vi "Make.vi"(8 "error in (no error)":errorcluster, 9 "Item Refnum":refnum<vi>, 10 "Target":refnum<vi>, 11 "Coupled Message Scripter":refnum<class "Coupled Message Scripter.lvclass">) -> (0 "error out":errorcluster, 3 "Coupled Message Scripter out":refnum<class "Coupled Message Scripter.lvclass">)   [LabVIEW 2020, in "Message Maker.lvlib" / "Coupled Message Scripter.lvclass"]
uses:
  Coupled Message Scripter.lvclass
  Coupled Message Scripter.lvclass/Coupled Message Scripter.ctl
  Message Maker.lvlib
  Message Scripter/Message Scripter.lvclass
  <vilib>/ErrorRing/Error Ring.xnode
  <vilib>/Utility/error.llb/Error Cluster From Error Code.vi
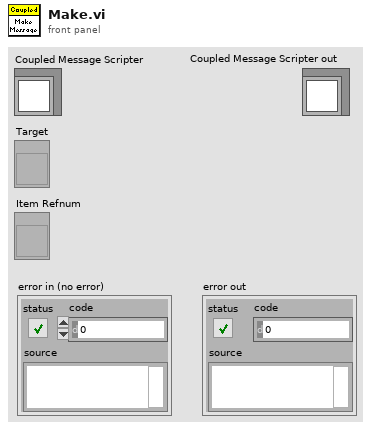
[diagram p1: front panel]
types:
  T1 = enum32{"invalid scope", "public", "private", "protected", "community"}
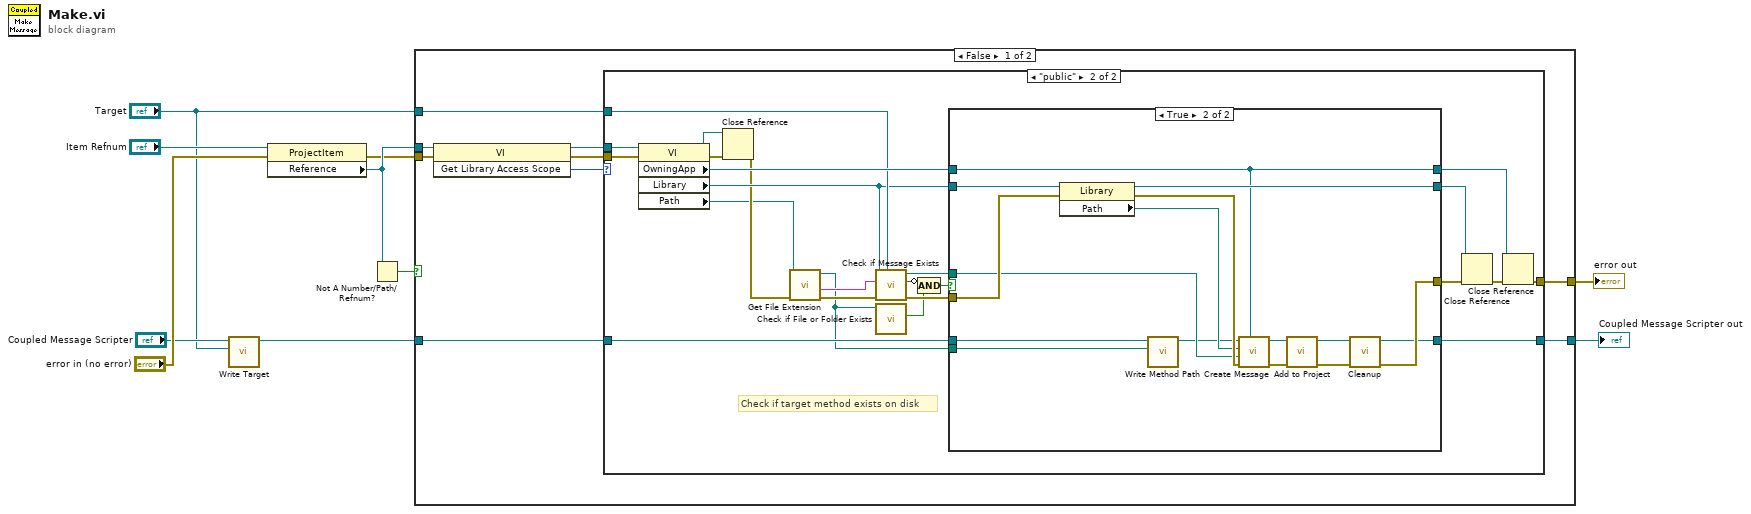
[diagram p0: block diagram]
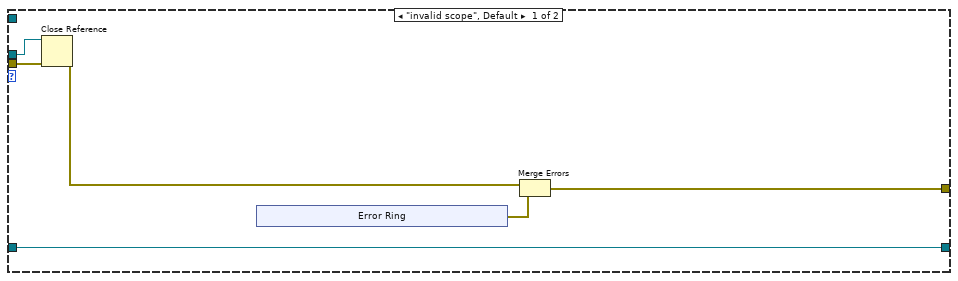
[diagram p2: hidden frame]
diagram:
  n1 = call "Write Target.vi"("Target"="Target", "Message Scripter in"="Coupled Message Scripter") -> ("Message Scripter out"=w2:refnum<class "Coupled Message Scripter.lvclass">)  [unwired: 9 in]
  n2 = property class="ProjectItem"(reference="Item Refnum", error in="error in (no error)") -> (error out=w6:errorcluster, "Reference"=w7:refnum<vi>)  [unwired: 1 out]
  n3 = Not A Number/Path/Refnum?(number/path/refnum=w7) -> (NaN/Path/Refnum?=w8:bool)
  n4 = case shown="False" w8 {
    tunnel: [w19 w76] -> w10
    tunnel: "Target" -> [w18 _]
    tunnel: w6 -> [w17 w76]
    tunnel: w7 -> [w16 _]
    tunnel: w2 -> [w12 w75]
    tunnel: [w11 w75] -> w9
    frame False {
      n5 = invoke class="VI" method="Get Library Access Scope"(reference=w16, error in=w17) -> (reference out=w15:refnum<vi>, error out=w14:errorcluster, "Get Library Access Scope"=w13:T1)  [unwired: 1 in]
      n6 = case shown="\"public\"" w13 {
        tunnel: [w21 w52] -> w19
        tunnel: w18 -> [_ w48]
        tunnel: w15 -> [w24 w42]
        tunnel: w14 -> [w25 w41]
        tunnel: w12 -> [w22 w40]
        tunnel: [w22 w39] -> w11
        frame "invalid scope", Default {
          n7 = Close Reference(reference=w24, error in (no error)=w25) -> (error out=w23:errorcluster)
          n8 = xnode "Error Ring"() -> ("error out"=w20:errorcluster)
          n9 = Merge Errors(w23, w20) -> (w21:errorcluster)
        }
        frame "public" {
          # "Check if target method exists on disk"
          n10 = property class="VI"(reference=w42, error in=w41) -> (reference out=w44:refnum<vi>, error out=w45:errorcluster, "OwningApp"=w50:refnum<vi>, "Library"=w46:refnum<vi>, "Path"=w35:path)
          n11 = Close Reference(reference=w44, error in (no error)=w45) -> (error out=w37:errorcluster)
          n12 = call <vilib>:"Get File Extension.vi"("error in (no error)"=w37, "file"=w35) -> ("error out"=w36:errorcluster, "filename without extension"=w38:string, "dup file"=w34:path)  [unwired: 5 in, 2 out]
          n13 = call "Check if Message Exists.vi"("Target"=w48, "error in (no error)"=w36, "Method Name"=w38, "Actor"=w46) -> ("error out"=w54:errorcluster, "Message Class Exists?"=w33:bool, "Message Path"=w49:path)  [unwired: 5 in]
          n14 = call <vilib>:"Check if File or Folder Exists.vi"("path"=w34) -> ("file or folder exists?"=w32:bool)  [unwired: 8 in, 2 out]
          n15 = Compound Arithmetic op=AND(invert w33, w32) -> (w31:bool)
          n16 = case shown="True" w31 {
            tunnel: w50 -> [w57 w69]
            tunnel: w49 -> [_ w68]
            tunnel: w54 -> [w58 w72]
            tunnel: [w58 w64] -> w51
            tunnel: [w57 w69] -> w47
            tunnel: w46 -> [w56 w73]
            tunnel: [w56 w70] -> w43
            tunnel: w40 -> [w55 w61]
            tunnel: [w55 w62] -> w39
            tunnel: w34 -> [_ w59]
            frame False {
            }
            frame True {
              n17 = property class="Library"(reference=w73, error in=w72) -> (reference out=w70:refnum<vi>, error out=w71:errorcluster, "Path"=w67:path)
              n18 = call "Write Method Path.vi"("Method Path"=w59, "Message Scripter in"=w61) -> ("Message Scripter out"=w60:refnum<class "Coupled Message Scripter.lvclass">)  [unwired: 9 in]
              n19 = call "Create Message.vi"("AppInst"=w69, "error in (no error)"=w71, "Destination Path"=w68, "Actor class path"=w67, "Message Maker in"=w60) -> ("error out"=w66:errorcluster, "Message Maker out"=w74:refnum<class "Coupled Message Scripter.lvclass">)  [unwired: 5 in]
              n20 = call-dynamic "Add to Project.vi"("error in (no error)"=w66, "Coupled Message Scripter in"=w74) -> ("error out"=w65:errorcluster, "Coupled Message Scripter out"=w63:refnum<class "Coupled Message Scripter.lvclass">)  [unwired: 8 in]
              n21 = call-dynamic "Cleanup.vi"("error in (no error)"=w65, "Message Scripter in"=w63) -> ("error out"=w64:errorcluster, "Message Scripter out"=w62:refnum<class "Coupled Message Scripter.lvclass">)  [unwired: 8 in]
            }
          }
          n22 = Close Reference(reference=w43, error in (no error)=w51) -> (error out=w53:errorcluster)
          n23 = Close Reference(reference=w47, error in (no error)=w53) -> (error out=w52:errorcluster)
        }
      }
    }
    frame True {
    }
  }
  "error out" <- w10
  "Coupled Message Scripter out" <- w9
